vi "PicoC_Mode.vi"(8 "error in (no error)":errorcluster, 10 "Enable?":bool, 11 "SRV In":refnum<k5>) -> (0 "error out":errorcluster, 3 "SRV Out":refnum<k5>)   [LabVIEW 2009]
doc: "Controls the Pico mode (on/off) based on the boolean input.\n\n\nModified for Benilde St. Margaret's School - Tim Jump\nBy Doug Schmertman - Logic PD\nCopyright 2012"
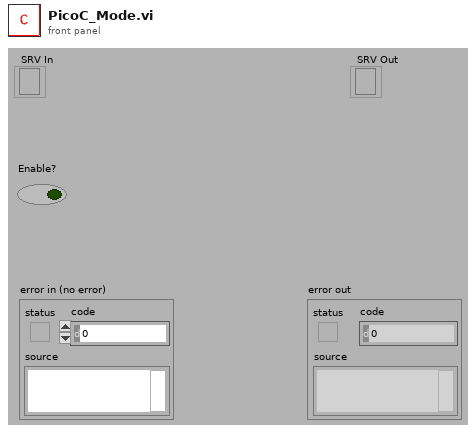
[diagram p1: front panel]
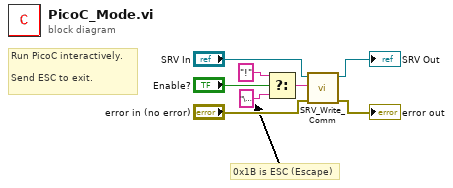
[diagram p0: block diagram]
diagram:
  # "Run PicoC interactively.\n\nSend ESC to exit."
  # "0x1B is ESC (Escape)"
  n1 = Select(t="!" ("Command Sent"), s="Enable?", f="\u001b" ("Text to send 2")) -> (s? t:f=w3:string)
  n2 = call "SRV_Write_Comm.vi"("error in (no error)"="error in (no error)", "Command Sent"=w3, "SRV In"="SRV In") -> ("error out"=→"error out":errorcluster, "SRV Out"=→"SRV Out":refnum<k5>)  [unwired: 6 in, 1 out]
